vi "串口上位机.vi"() -> ()   [LabVIEW 2013]
uses:
  <vilib>/Instr/_visa.llb/VISA Flush IO Buffer Mask.ctl
  <vilib>/Instr/_visa.llb/VISA Configure Serial Port (Instr).vi
panel:
  in  "命令":string="*IDN?"
  in  "发送":bool
  out "当前温度":dbl(slide) scale=0.0..100.0
  out "当前温度":dbl
  out "报警灯":bool
  out "温度波形图":T1(graph)
  in  "温度最低限定值":dbl
  in  "温度最高限定值":dbl
  out "表格实际路径":path
  in  "文件路径（基路径）":path
  out "读取缓冲区":string
  in  "停止":bool
  in  "VISA资源名称":refnum<visa-resource-name>="COM1"
  in  "串口基本配置":T2={"波特率"=9600, "数据比特"=8, "奇偶"=enum."None", "停止位"=10, "流控制"=0, "termination char\n(0xA = '\\n' = LF) "=10} {"termination char\n(0xA = '\\n' = LF)" format="%.0x"; "流控制" items=["无"=0, "XON/XOFF"=1, "RTS/CTS"=2, "DTR/DSR"=4]; "停止位" items=["1.0"=10, "1.5"=15, "2.0"=20]; "数据比特" min=5 max=8 step=1; "波特率" items=["75"=75, "110"=110, "134"=134, "150"=150, "300"=300, "600"=600, "1200"=1200, "1800"=1800, "2400"=2400, "4800"=4800, "7200"=7200, "9600"=9600, "14400"=14400, "19200"=19200, "28800"=28800, "38400"=38400, "56000"=56000, "57600"=57600, "115200"=115200, "128000"=128000, "230400"=230400]}
  # "自动售餐机监控平台"
  # "软件使用说明：\n1.先将单片机连好电脑，设置好串口参数，点击开始运行。\n2.温度检测：先设置好温度的范围值，再打开Start键\n3.销售明细：每接收一次生成一个excel表格。请在接收之前定义好表格所在的基路径\n：如D：\\file。实际则会在D：\\file生成.xls文件\n4.单片机发送数据格式：\n销售明细：'m'+数据+‘\\n’\n温度上传：'t'+数据+‘\\n’\n5.发送给单片机:  's'+xx(最低温度)+jj(最高温度)+回车\n5.上位机控制单片机：发送's'+xx,+xx   (第二个字符表示最低温度，第三个字符表示最高温度)"
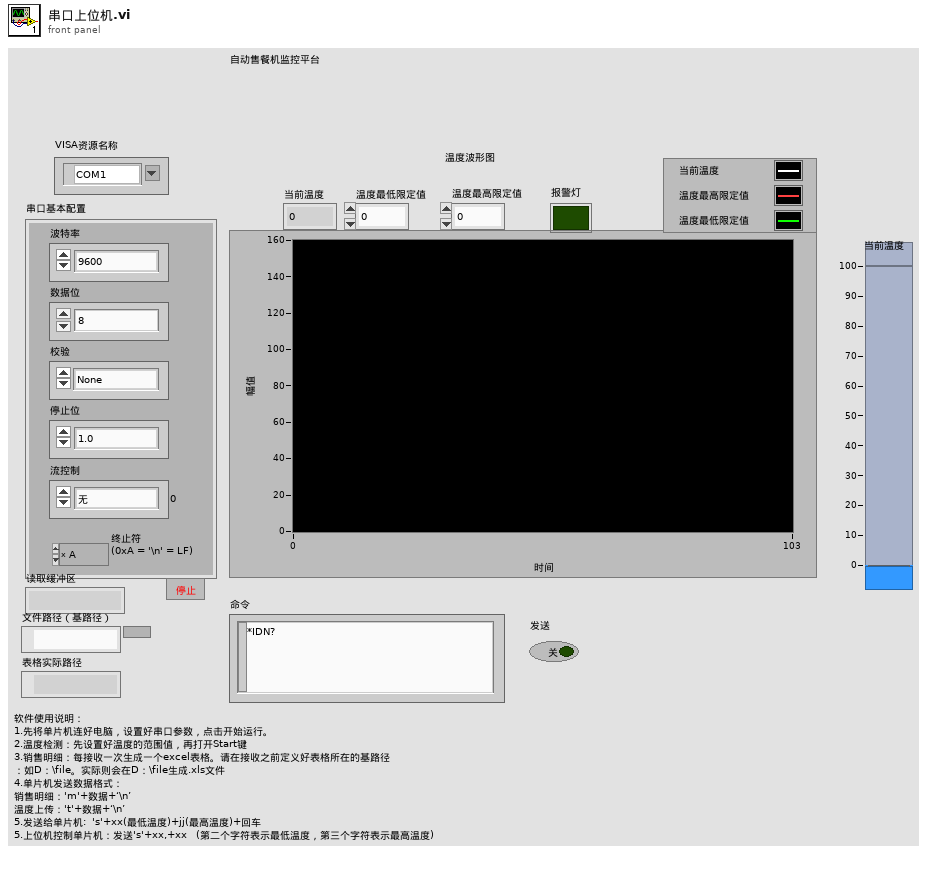
[diagram p1: front panel]
types:
  T1 = cluster{"当前温度":dbl, "温度最高限定值":dbl, "温度最低限定值":dbl}
  T2 = cluster{"波特率":u32, "数据比特":u16, "奇偶":enum16{"None", "Odd", "Even", "Mark", "Space"}, "停止位":u16, "流控制":u16, "termination char\n(0xA = '\\n' = LF) ":u8}
  T3 = typedef "VISA Flush IO Buffer Mask.ctl" = u16
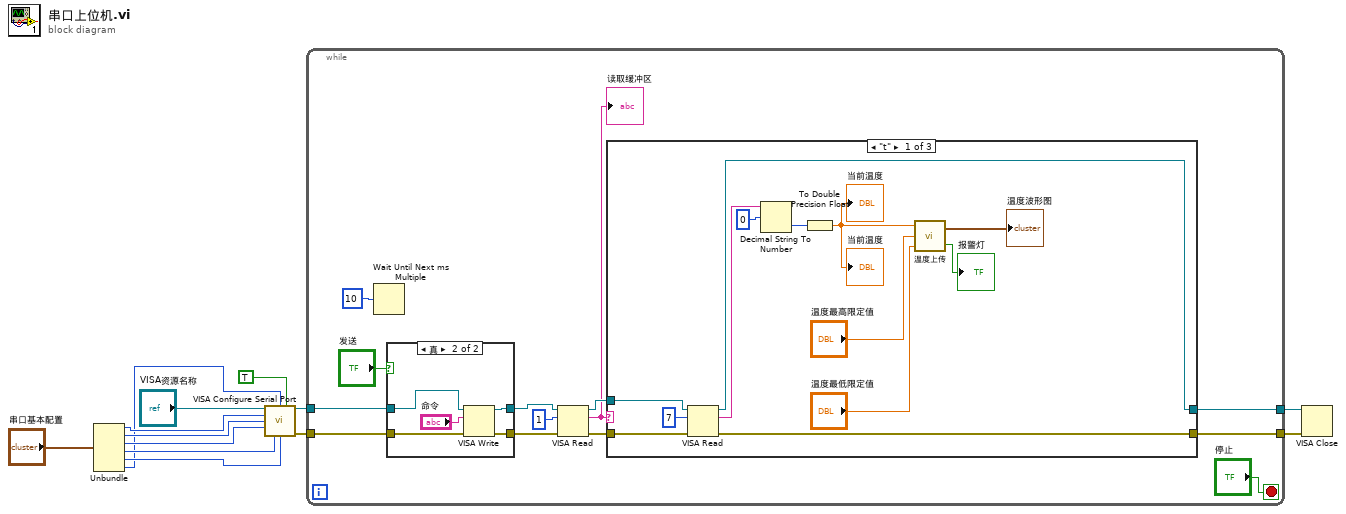
[diagram p0: block diagram]
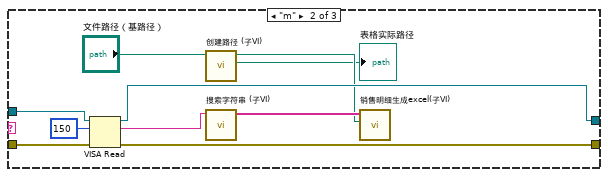
[diagram p3: hidden frame]
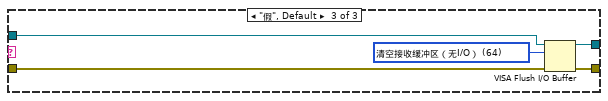
[diagram p4: hidden frame]
diagram:
  n1 = Unbundle("串口基本配置") -> ("波特率"=w11:u32, "数据比特"=w10:u16, "奇偶"=w9:enum16{"None", "Odd", "Even", "Mark", "Space"}, "停止位"=w8:u16, "流控制"=w7:u16, "termination char\n(0xA = '\\n' = LF)"=w3:u8)
  n2 = call-poly "VISA Configure Serial Port"("VISA resource name"="VISA资源名称", "termination char\n(0xA = '\\n' = LF)"=w3, "Enable Termination\nChar (T)"=TRUE ("Enable Termination\nChar (T)"), "baud rate (9600)"=w11, "data bits (8)"=w10, "parity (0:none)"=w9, "stop bits (10: 1 bit)"=w8, "flow control (0:none)"=w7) -> ("VISA resource name out"=w2:refnum<visa-resource-name>, "error out"=w1:errorcluster)  [unwired: 6 in]
  n3 = while {
    tunnel: [w22] -> w6
    tunnel: [w20] -> w5
    tunnel: w2 -> [w18]
    tunnel: w1 -> [w17]
    stop <- "停止" stop-if-true
    n4 = Wait Until Next ms Multiple(millisecond multiple=u32 10 ("毫秒倍数")) -> ()  [unwired: 1 out]
    n5 = case shown="真" "发送" {
      tunnel: w18 -> [w28 w33]
      tunnel: w17 -> [w27 w32]
      tunnel: [w28 w31] -> w15
      tunnel: [w27 w30] -> w14
      frame False {
      }
      frame True {
        n6 = VISA Write(VISA resource name=w33, write buffer="命令", error in (no error)=w32) -> (VISA resource name out=w31:refnum<visa-resource-name>, error out=w30:errorcluster)  [unwired: 1 out]
      }
    }
    n7 = VISA Read(VISA resource name=w15, byte count=u32 1 ("字节总数"), error in (no error)=w14) -> (VISA resource name out=w25:refnum<visa-resource-name>, read buffer=w19:string, error out=w24:errorcluster)  [unwired: 1 out]
    "读取缓冲区" <- w19
    n8 = case shown="\"t\"" w19 {
      tunnel: w25 -> [w46 w56 w61]
      tunnel: w24 -> [w44 w55 w60]
      tunnel: [w43 w54 w59] -> w22
      tunnel: [w42 w53 w58] -> w20
      frame "t" {
        n9 = VISA Read(VISA resource name=w46, byte count=u32 7 ("字节总数"), error in (no error)=w44) -> (VISA resource name out=w43:refnum<visa-resource-name>, read buffer=w41:string, error out=w42:errorcluster)  [unwired: 1 out]
        n10 = Decimal String To Number(string=w41, offset=0 ("偏移量")) -> (number=w39:i32)  [unwired: 1 in, 1 out]
        n11 = To Double Precision Float(number=w39) -> (double precision float=w34:dbl)
        "当前温度" <- w34
        "当前温度" <- w34
        n12 = call "温度上传.vi"("温度最低限定值"="温度最低限定值", "温度最高限定值"="温度最高限定值", "当前温度"=w34) -> ("报警灯"=→"报警灯":bool, "温度曲线"=→"温度波形图":T1)
      }
      frame "m" {
        n13 = VISA Read(VISA resource name=w56, byte count=u32 150 ("字节总数"), error in (no error)=w55) -> (VISA resource name out=w54:refnum<visa-resource-name>, read buffer=w51:string, error out=w53:errorcluster)  [unwired: 1 out]
        n14 = call "创建路径 (子VI).vi"("文件路径（基路径）"="文件路径（基路径）") -> ("表格实际路径"=→"表格实际路径":path, "appended path"=w49:path)  [unwired: 9 in]
        n15 = call "搜索字符串 (子VI).vi"("read buffer"=w51) -> ("数组"=w50:string[])  [unwired: 10 in]
        n16 = call "销售明细生成excel(子VI).vi"("appended path"=w49, "数组"=w50) -> ()  [unwired: 10 in]
      }
      frame "假", Default {
        w57 = T3 64 items=["清空接收缓冲区"=16, "向设备写入传输缓冲区"=32, "清空接收缓冲区（无I/O）"=64, "清空传输缓冲区"=128] ("Mask")
        n17 = VISA Flush I/O Buffer(VISA resource name=w61, mask (16)=w57, error in (no error)=w60) -> (VISA resource name out=w59:refnum<visa-resource-name>, error out=w58:errorcluster)
      }
    }
  }
  n18 = VISA Close(VISA resource name=w6, error in (no error)=w5) -> ()  [unwired: 1 out]
